vi "SuperNS_CreateWithContext.vi"(0 "reference in":refnum<class "SuperNS.lvclass">, 1 "Writer (F: Reader)":bool, 2 "Local EP Config":cluster{"Context":string, "Name":string}, 3 "Remote EP Config":T3, 4 "Connection Config":T2={"BufferSize (100)"=100, "Connection Lost Timeout (2000 ms)"=2000, "Element Allocation Mode"=0, "Low latency mode"=enum."None (High througput mode)", "BG ConnCheck/Read period (200 ms)"=200, "OpenProcessWindow(F)"=FALSE} {"Element Allocation Mode" items=["allocate as needed", "pre-allocate"]}, 5 "error in (no error)":errorcluster) -> (14 "reference out":refnum<class "SuperNS.lvclass">, 19 "error out":errorcluster)   [LabVIEW 2020, in "SuperNS.lvclass"]
doc: "Copyright © 2008 - 2024 VI Technologies B.V. \nALL RIGHTS RESERVED\n\n<b>Instantiates a SuperNS object.</b>\n\nDepending on the Writer input, internally creates the reader or writer endpoint of a network stream. The stream is of type LabVIEW Object (flattened to string).\n\nBy using this create you to have the possibility to use connect to a SuperNS endpoint on the local host. Using a context definition enables this. \n\nA SuperNS is an active object. It has a background process for stream (re)connecting and data reading.\n\nYou must always wire the <b>Local EP Config</b> input and all its string inputs must be filled. \n\nYou should wire the <b>Remote EP Config</b> on only one of the endpoints to point to the other endpoint. The string input fields of the <b>Remote EP Config</b> cluster must filled strings for all fields when defining the endpoint. To use the <b>Localhost</b> as IP, write \"localhost\" to the IP field.\n\nThe <b>Context</b> field of the <b>Local EP Config</b> and <b>Remote EP Config</b> are not allowed to be equal.\n\nCall the <b>GetReadDataEventRef</b> method to get an event registration refnum which you can use to retrieve the read data (for a reader endpoint) in an event structure.\n\nCall <b>WriteToStream</b> to write data to the stream (for a writer endpoint)\n\nSet <b>Connection Config.OpenProcessWindow</b> input to true if you want to see the background process' frontpanel. You can always show/hide it at runtime by calling <b>OpenCloseThreadWin</b> method.\n\nAll other inputs are passed through to the network stream functions. See the LabVIEW help for more information on these.\n\nCall the <b>Destroy</b> method to destroy the object (and the network stream endpoint contained within).\n\nRefer to the Streaming Data and Sending Commands between Applications LabVIEW help topic for more information about using network streams."
uses:
  SuperNS.lvclass
  <vilib>/dex/Stream Element Allocation Mode.ctl
  <vilib>/Utility/error.llb/Error Cluster From Error Code.vi
  <vilib>/ErrorRing/Error Ring.xnode
  SuperNS.lvclass/SuperNS.ctl
panel:
  # "Copyright (c) 2024, VI Technologies B.V.\nAll rights reserved.\n\nRedistribution and use in source and binary forms, with or without modification, are permitted provided that \nthe following conditions are met:\n\n * Redistributions of source code must retain the above copyright notice, this list of conditions and the \nfollowing disclaimer.\n * Redistributions in binary form must reproduce the above copyright notice, this list of conditions and the \nfollowing disclaimer in the documentation and/or other materials provided with the distribution.\n * Neither the name of VI Technologies B.V. nor the names of its contributors may be used to endorse or \npromote products derived from this software without specific prior written permission.\n\nTHIS SOFTWARE IS PROVIDED BY THE COPYRIGHT HOLDERS AND CONTRIBUTORS \"AS IS\" AND ANY EXPRESS OR \nIMPLIED WARRANTIES, INCLUDING, BUT NOT LIMITED TO, THE IMPLIED WARRANTIES OF MERCHANTABILITY \nAND FITNESS FOR A PARTICULAR PURPOSE ARE DISCLAIMED. IN NO EVENT SHALL THE COPYRIGHT OWNER OR \nCONTRIBUTORS BE LIABLE FOR ANY DIRECT, INDIRECT, INCIDENTAL, SPECIAL, EXEMPLARY, OR CONSEQUENTIAL \nDAMAGES (INCLUDING, BUT NOT LIMITED TO, PROCUREMENT OF SUBSTITUTE GOODS OR SERVICES; LOSS OF \nUSE, DATA, OR PROFITS; OR BUSINESS INTERRUPTION) HOWEVER CAUSED AND ON ANY THEORY OF LIABILITY, \nWHETHER IN CONTRACT, STRICT LIABILITY, OR TORT (INCLUDING NEGLIGENCE OR OTHERWISE) ARISING IN ANY \nWAY OUT OF THE USE OF THIS SOFTWARE, EVEN IF ADVISED OF THE POSSIBILITY OF SUCH DAMAGE.\n\nFor more information, please visit https://www.vi-tech.nl or contact us at info@vi-tech.nl"
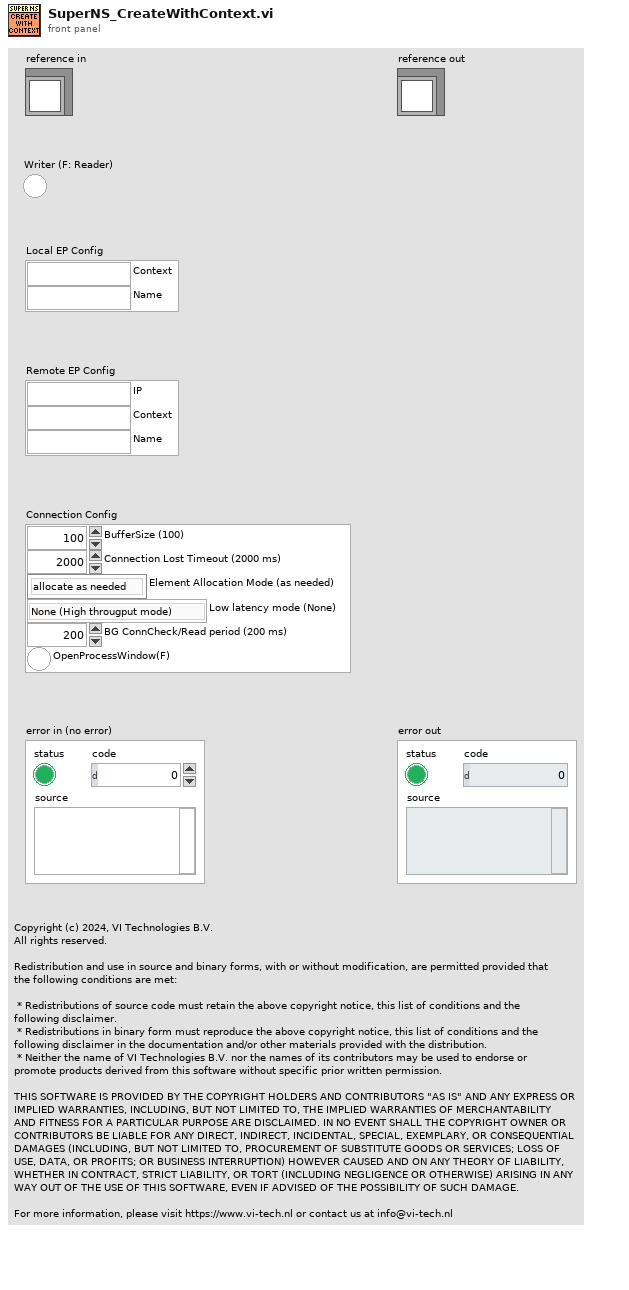
[diagram p1: front panel]
types:
  T1 = typedef "Stream Element Allocation Mode.ctl" = u32
  T2 = cluster{"BufferSize (100)":i32, "Connection Lost Timeout (2000 ms)":i32, "Element Allocation Mode":T1, "Low latency mode":enum16{"None (High througput mode)", "All Elements Read From Stream", "All Elements Available for Reading"}, "BG ConnCheck/Read period (200 ms)":i32, "OpenProcessWindow(F)":bool}
  T3 = cluster{"IP":string, "Context":string, "Name":string}
  T4 = enum16{"None (High througput mode)", "All Elements Read From Stream", "All Elements Available for Reading"}
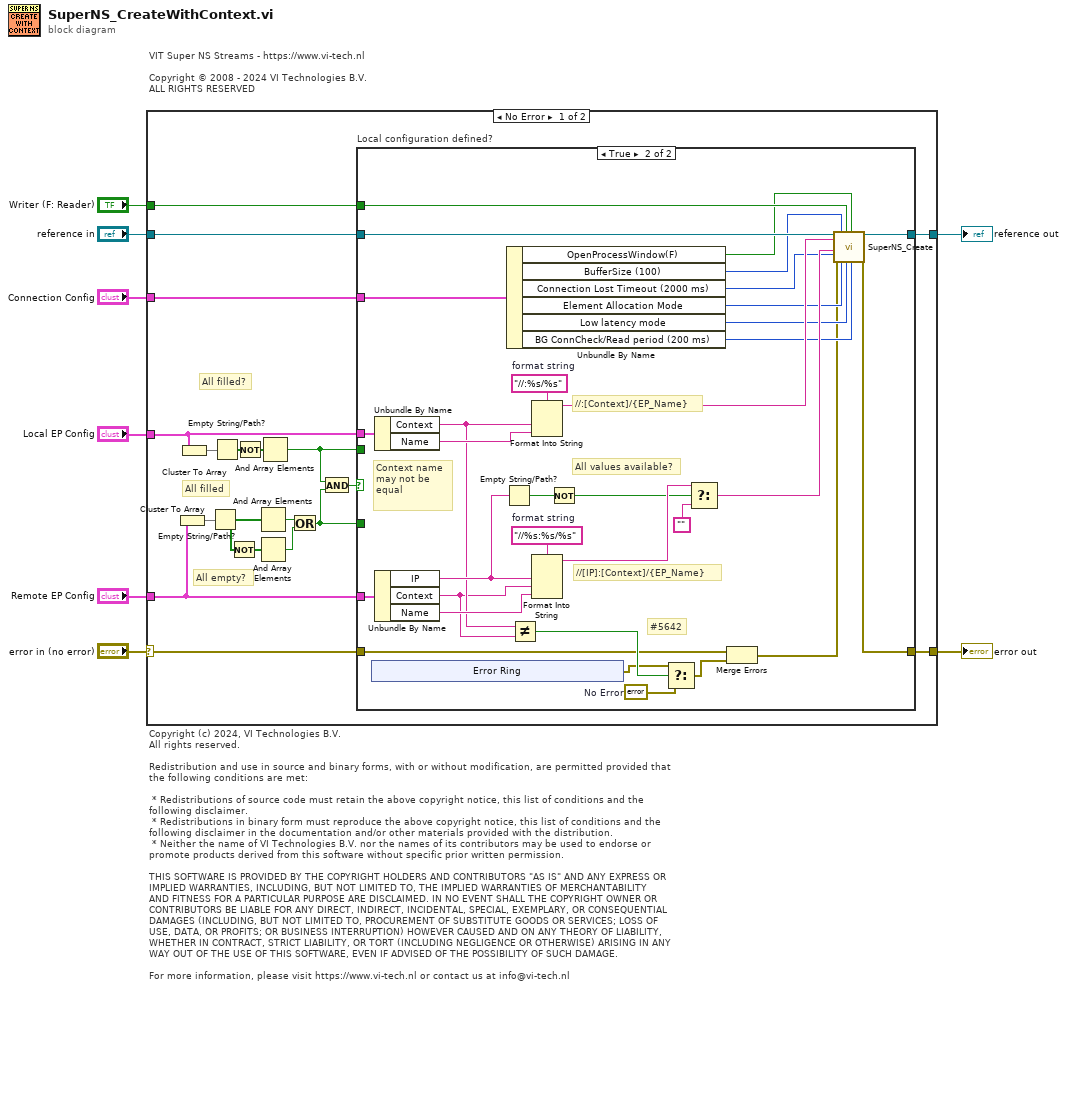
[diagram p0: block diagram]
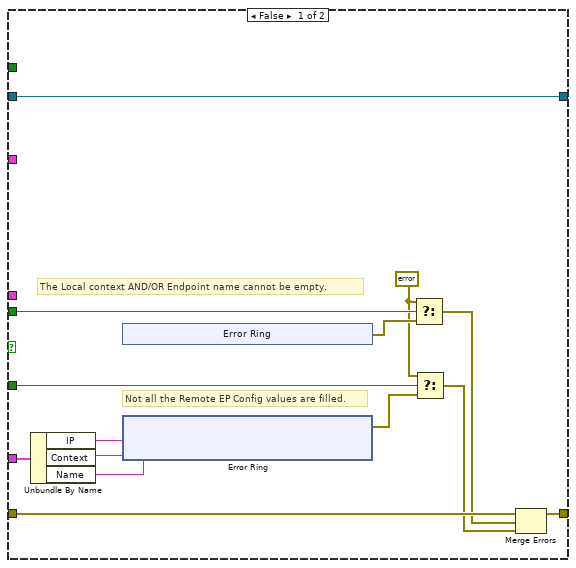
[diagram p2: hidden frame]
diagram:
  # "VIT Super NS Streams - https://www.vi-tech.nl\n\nCopyright © 2008 - 2024 VI Technologies B.V. \nALL RIGHTS RESERVED"
  # "Copyright (c) 2024, VI Technologies B.V.\nAll rights reserved.\n\nRedistribution and use in source and binary forms, with or without modification, are permitted provided that \nthe following conditions are met:\n\n * Redistributions of source code must retain the above copyright notice, this list of conditions and the \nfollowing disclaimer.\n * Redistributions in binary form must reproduce the above copyright notice, this list of conditions and the \nfollowing disclaimer in the documentation and/or other materials provided with the distribution.\n * Neither the name of VI Technologies B.V. nor the names of its contributors may be used to endorse or \npromote products derived from this software without specific prior written permission.\n\nTHIS SOFTWARE IS PROVIDED BY THE COPYRIGHT HOLDERS AND CONTRIBUTORS \"AS IS\" AND ANY EXPRESS OR \nIMPLIED WARRANTIES, INCLUDING, BUT NOT LIMITED TO, THE IMPLIED WARRANTIES OF MERCHANTABILITY \nAND FITNESS FOR A PARTICULAR PURPOSE ARE DISCLAIMED. IN NO EVENT SHALL THE COPYRIGHT OWNER OR \nCONTRIBUTORS BE LIABLE FOR ANY DIRECT, INDIRECT, INCIDENTAL, SPECIAL, EXEMPLARY, OR CONSEQUENTIAL \nDAMAGES (INCLUDING, BUT NOT LIMITED TO, PROCUREMENT OF SUBSTITUTE GOODS OR SERVICES; LOSS OF \nUSE, DATA, OR PROFITS; OR BUSINESS INTERRUPTION) HOWEVER CAUSED AND ON ANY THEORY OF LIABILITY, \nWHETHER IN CONTRACT, STRICT LIABILITY, OR TORT (INCLUDING NEGLIGENCE OR OTHERWISE) ARISING IN ANY \nWAY OUT OF THE USE OF THIS SOFTWARE, EVEN IF ADVISED OF THE POSSIBILITY OF SUCH DAMAGE.\n\nFor more information, please visit https://www.vi-tech.nl or contact us at info@vi-tech.nl"
  n1 = case shown="No Error" "error in (no error)" {
    selector: "error in (no error)" -> [w21 w94]
    tunnel: [w22 w94] -> w1
    tunnel: [w23 w93] -> w7
    tunnel: "reference in" -> [w24 w93]
    tunnel: "Local EP Config" -> [w25 _]
    tunnel: "Remote EP Config" -> [w19 _]
    tunnel: "Connection Config" -> [w9 _]
    tunnel: "Writer (F: Reader)" -> [w10 _]
    frame No Error {
      # "All empty?"
      # "All filled"
      # "All filled?"
      n2 = Cluster To Array(cluster=w19) -> (array=w20:string[])
      n3 = Cluster To Array(cluster=w25) -> (array=w26:string[])
      n4 = Empty String/Path?(string/path=w20) -> (empty?=w16:bool[])
      n5 = Empty String/Path?(string/path=w26) -> (empty?=w27:bool[])
      n6 = Not(x=w16) -> (.not. x?=w18:bool[])
      n7 = Not(x=w27) -> (.not. x?=w11:bool[])
      n8 = And Array Elements(Boolean array=w16) -> (logical AND=w15:bool)
      n9 = And Array Elements(Boolean array=w18) -> (logical AND=w17:bool)
      n10 = And Array Elements(Boolean array=w11) -> (logical AND=w13:bool)
      n11 = Or(x=w15, y=w17) -> (x .or. y?=w12:bool)
      n12 = And(x=w13, y=w12) -> (x .and. y?=w14:bool)
      n13 = case "Local configuration defined?" shown="True" w14 {
        tunnel: w19 -> [w31 w78]
        tunnel: w25 -> [_ w87]
        tunnel: w24 -> [w41 w85]
        tunnel: [w41 w84] -> w23
        tunnel: [w40 w83] -> w22
        tunnel: w21 -> [w39 w60]
        tunnel: w13 -> [w38 _]
        tunnel: w12 -> [w35 _]
        tunnel: w10 -> [_ w77]
        tunnel: w9 -> [_ w56]
        frame False {
          w34 = errorcluster {"status"=FALSE, "code"=0, "source"=""} ("t")
          # "The Local context AND/OR Endpoint name cannot be empty."
          # "Not all the Remote EP Config values are filled."
          n14 = Unbundle By Name(w31) -> ("IP"=w30:string, "Context"=w29:string, "Name"=w28:string)
          n15 = xnode "Error Ring"() -> ("error out"=w37:errorcluster)
          n16 = xnode "Error Ring"("parameter 0"=w30, "parameter 1"=w29, "parameter 2"=w28) -> ("error out"=w33:errorcluster)
          n17 = Select(t=w34, s=w38, f=w37) -> (s? t:f=w36:errorcluster)
          n18 = Select(t=w34, s=w35, f=w33) -> (s? t:f=w32:errorcluster)
          n19 = Merge Errors(w39, w36, w32) -> (w40:errorcluster)
        }
        frame True {
          w57 = errorcluster {"status"=FALSE, "code"=0, "source"=""}  # No Error
          w74 = "//%s:%s/%s"  # format string
          w76 = "//:%s/%s"  # format string
          # "#5642"
          # "All values available?"
          # "//[IP]:[Context]/{EP_Name}"
          # "//:[Context]/{EP_Name}"
          # "Context name\nmay not be equal"
          n20 = xnode "Error Ring"() -> ("error out"=w61:errorcluster)
          n21 = Unbundle By Name(w87) -> ("Context"=w80:string, "Name"=w86:string)
          n22 = Unbundle By Name(w78) -> ("IP"=w82:string, "Context"=w79:string, "Name"=w81:string)
          n23 = Empty String/Path?(string/path=w82) -> (empty?=w69:bool)
          n24 = Unbundle By Name(w56) -> ("OpenProcessWindow(F)"=w67:bool, "BufferSize (100)"=w68:i32, "Connection Lost Timeout (2000 ms)"=w66:i32, "Element Allocation Mode"=w65:T1, "Low latency mode"=w64:T4, "BG ConnCheck/Read period (200 ms)"=w63:i32)
          n25 = Not Equal?(x=w80, y=w79) -> (x != y?=w62:bool)
          n26 = Format Into String(format string=w76, w80, w86) -> (resulting string=w75:string)  [unwired: 2 in, 1 out]
          n27 = Format Into String(format string=w74, w82, w79, w81) -> (resulting string=w72:string)  [unwired: 2 in, 1 out]
          n28 = Not(x=w69) -> (.not. x?=w70:bool)
          n29 = Select(t=w61, s=w62, f=w57) -> (s? t:f=w58:errorcluster)
          n30 = Select(t=w72, s=w70, f="") -> (s? t:f=w73:string)
          n31 = Merge Errors(w60, w58) -> (w59:errorcluster)
          n32 = call "SuperNS_Create.vi"("reference in"=w85, "NSName"=w75, "RemoteEP_URL"=w73, "Connection Lost Timeout (2000 ms)"=w66, "error in (no error)"=w59, "BufferSize (100)"=w68, "Element Allocation Mode"=w65, "Writer (F: Reader)"=w77, "Low latency mode"=w64, "OpenProcessWindow(F)"=w67, "BG ConnCheck/Read period (200 ms)"=w63) -> ("SuperNS Reference"=w84:refnum<class "SuperNS.lvclass">, "error out"=w83:errorcluster)  [unwired: 7 in]
        }
      }
    }
    frame Error {
    }
  }
  "reference out" <- w7
  "error out" <- w1
